vi "Sequence - Define Test Equipment.vi"(8 "error in (no error)":errorcluster) -> (0 "error out":errorcluster)   [LabVIEW 2020]
uses:
  Library - Test Executive.llb/Test Executive - Globals.vi
  Library - Test Executive.llb/Test Executive.lvlib
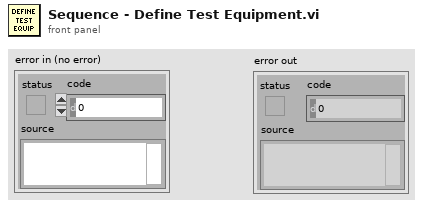
[diagram p1: front panel]
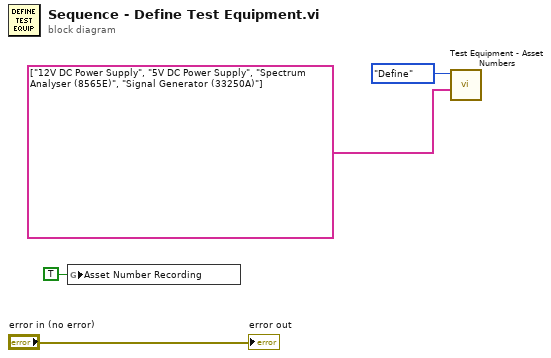
[diagram p0: block diagram]
diagram:
  n1 = global write "Test Executive - Globals.vi" "Asset Number Recording"(TRUE ("Asset Number Recording")) -> ()
  n2 = call "Test Equipment - Asset Numbers.vi"("Test Equipment"=string[] ["12V DC Power Supply", "5V DC Power Supply", "Spectrum Analyser (8565E)", "Signal Generator (33250A)"], "Mode"=enum16{"Edit", "Define", "Load", "Save", "CSV"}."Define") -> ()  [unwired: 8 in, 2 out]
  "error out" <- "error in (no error)"
